vi "sine profile generation.vi"(0 "frequency":dbl=1.0 format="%0.2p", 1 "amplitude in degrees":dbl=20.0 format="%0.2p", 5 "sample frequency":dbl=1000.0) -> (2 "Array 2":i16[](array[numeric]), 3 "Array":bool[](array[boolean]), 4 "sample frequency 2":dbl, 6 "Direction Pulse Array":i16[](array[numeric]), 7 "Direction Pulse Graph":i16[](graph), 8 "Clock Pulse Boolean Array":bool[](array[boolean]), 9 "Clock Pulse Array":i32[](array[numeric]), 10 "Clock Pulse Graph":i32[](graph))   [LabVIEW 2009]
uses:
  <vilib>/measure/NI_MABase.lvlib
panel:
  out "missing steps":bool
  out "size(s)":i32
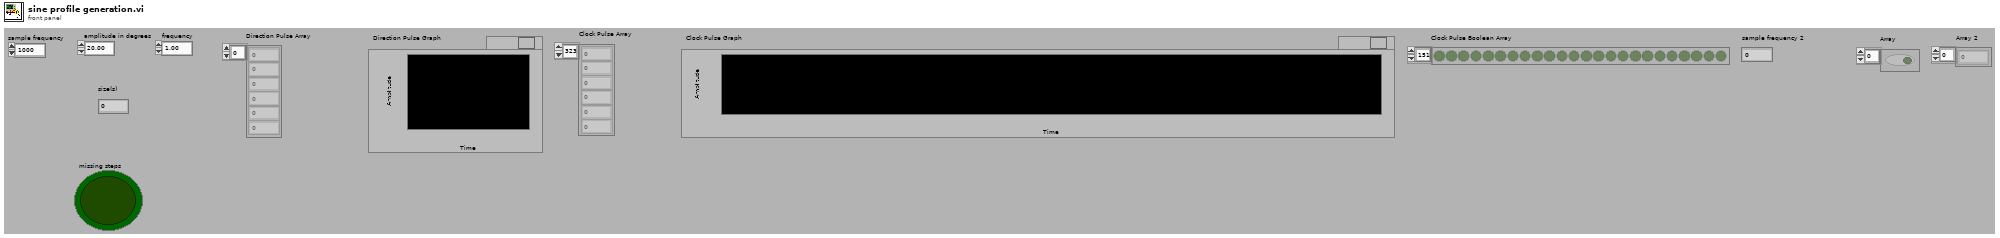
[diagram p1: front panel]
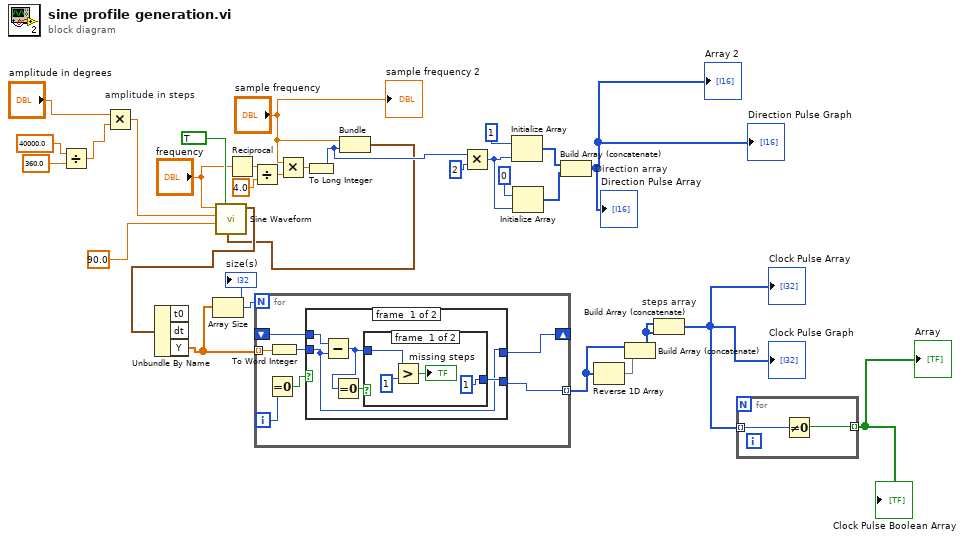
[diagram p0: block diagram]
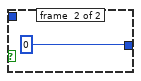
[diagram p2: hidden frame]
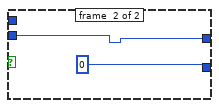
[diagram p3: hidden frame]
diagram:
  n1 = Divide(x=40000.0 ("y"), y=360.0) -> (x/y=w10:dbl)
  n2 = Multiply "amplitude in steps"(x="amplitude in degrees", y=w10) -> (x*y=w7:dbl)
  n3 = Reciprocal(x="frequency") -> (1/x=w11:dbl)
  n4 = Divide(x=w11, y=4.0) -> (x/y=w13:dbl)
  n5 = Multiply(x="sample frequency", y=w13) -> (x*y=w14:dbl)
  n6 = To Long Integer(number=w14) -> (32bit integer=w19:i32)
  n7 = Bundle("sample frequency"="sample frequency", w19) -> (w15:cluster{"sample frequency":dbl, i32})  [unwired: 1 in]
  n8 = call <vilib>:"Sine Waveform.vi"("sampling info"=w15, "reset signal"=TRUE, "phase"=90.0, "amplitude"=w7, "frequency"="frequency") -> ("signal out"=w28:waveform(dbl))  [unwired: 5 in, 1 out]
  n9 = Unbundle By Name(w28) -> ("Y"=w16:dbl[])  [unwired: 2 out]
  n10 = Array Size(array=w16) -> (size(s)=w26:i32)
  "size(s)" <- w26
  n11 = for {
    N: w26 -> [_]
    tunnel: w16 -> [w35] mode=indexing
    shift-right: [w31] -> _
    shift-left: _ -> [w33]
    tunnel: [w32] -> w27 mode=indexing
    i -> [w37]
    n12 = Equal To 0?(x=w37) -> (x = 0?=w36:bool)
    n13 = To Word Integer(number=w35) -> (16bit integer=w34:i16)
    n14 = case shown="False" w36 {
      tunnel: [w41 w49] -> w31
      tunnel: w34 -> [w41 w49]
      tunnel: w33 -> [w40 _]
      tunnel: [w42 0] -> w32
      frame #0 {
        n15 = Subtract(x=w40, y=w41) -> (x-y=w38:i16)
        n16 = Equal To 0?(x=w38) -> (x = 0?=w39:bool)
        n17 = case shown="False" w39 {
          tunnel: [1 0] -> w42
          tunnel: w38 -> [w45 _]
          frame #0 {
            n18 = Greater?(x=w45, y=1) -> (0:→"missing steps":bool)
          }
          frame #1 {
          }
        }
      }
      frame #1 {
      }
    }
  }
  n19 = Multiply(x=w19, y=2) -> (x*y=w22:i32)
  n20 = Initialize Array(i16 1 ("element"), w22) -> (w24:i16[])
  n21 = Initialize Array(i16 0 ("element"), w22) -> (w25:i16[])
  n22 = Build Array (concatenate) "Direction array"(w24, w25) -> (→"Direction Pulse Array" →"Direction Pulse Graph" →"Array 2":i16[])
  n23 = Reverse 1D Array(array=w27) -> (reversed array=w17:i32[])
  n24 = Build Array (concatenate)(w27, w17) -> (w18:i32[])
  n25 = Build Array (concatenate) "steps array"(w18, w18) -> (w2:i32[])
  "Clock Pulse Array" <- w2
  "Clock Pulse Graph" <- w2
  n26 = for {
    tunnel: w2 -> [w51] mode=indexing
    tunnel: [w50] -> w29 mode=indexing
    n27 = Not Equal To 0?(x=w51) -> (x != 0?=w50:bool)
  }
  "Clock Pulse Boolean Array" <- w29
  "Array" <- w29
  "sample frequency 2" <- "sample frequency"
